vi "COMI ENC Config.vi"(7 "bResetByZ":i32, 9 "mode":i32, 10 "ch":i32, 11 "hDevice":u32) -> (3 "hDevice out":u32)   [LabVIEW 2017, in "Comidll.lvlib"]
doc: "void (COMI_ENC_Config) (HANDLE hDevice, int ch, int mode, int bResetByZ);"
uses:
  <userlib>/Comidll/Comidll.lvlib
  <userlib>/Comidll/Comidll.dll
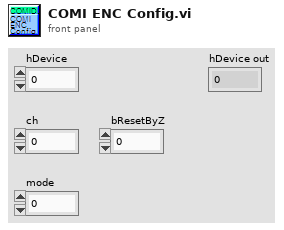
[diagram p1: front panel]
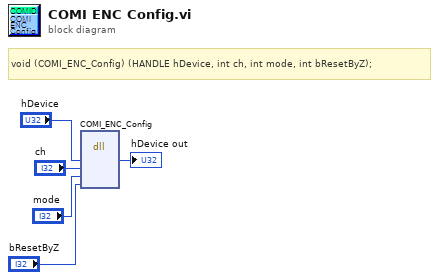
[diagram p0: block diagram]
diagram:
  # "void\t(COMI_ENC_Config) (HANDLE hDevice, int ch, int mode, int bResetByZ);"
  n1 = dll-call lib="C:/Program Files/National Instruments/LabVIEW 2017/user.lib/Comidll/Comidll.*" fn="COMI_ENC_Config"("hDevice"="hDevice", "ch"="ch", "mode"="mode", "bResetByZ"="bResetByZ") -> ("hDevice"=→"hDevice out":u32)  [unwired: 7 in, 2 out]
